vi "refreshElements.vi"(8 "error in (no error)":errorcluster, 9 "settingsFrontEndEvents":T1, 10 "Tab ref in":refnum<vi>) -> (0 "error out":errorcluster, 2 "Tab ref out":refnum<vi>)   [LabVIEW 2009, in "Views.lvlib" / "Camera.lvlib" / "andorSettingsViewer.lvclass"]
uses:
  andorSettingsViewer.lvclass
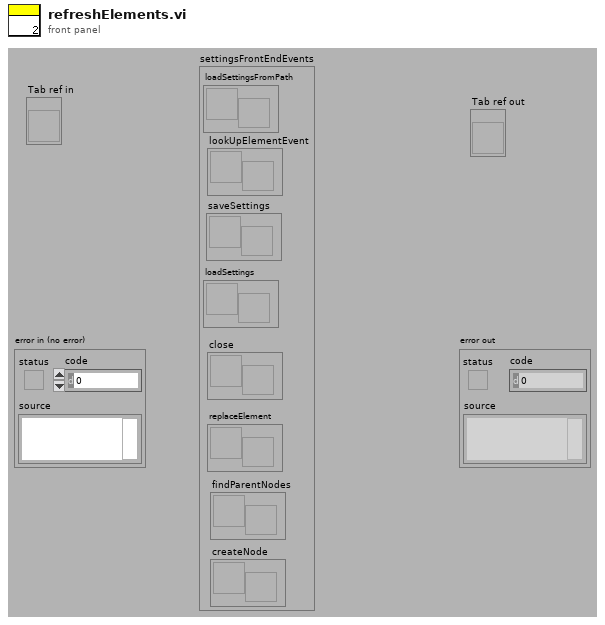
[diagram p1: front panel]
types:
  T1 = cluster{"loadSettingsFromPath":refnum<user-event>, "lookUpElementEvent":refnum<user-event>, "saveSettings":refnum<user-event>, "loadSettings":refnum<user-event>, "close":refnum<user-event>, "replaceElement":refnum<user-event>, "findParentNodes":refnum<user-event>, "createNode":refnum<user-event>}
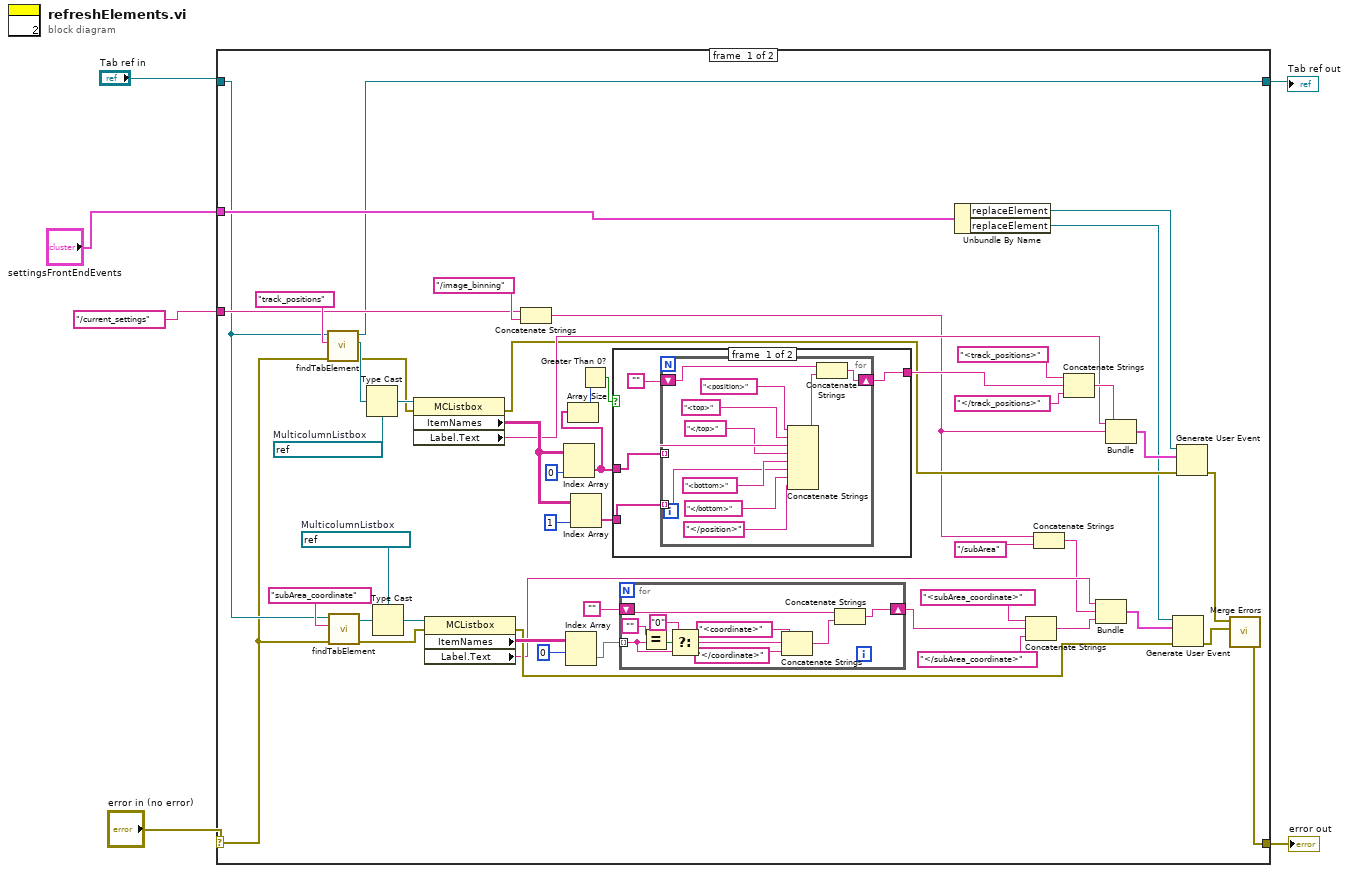
[diagram p0: block diagram]
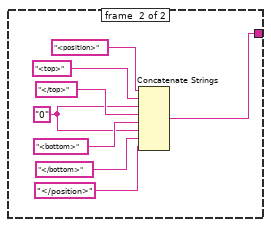
[diagram p2: hidden frame]
diagram:
  n1 = case shown="No Error" "error in (no error)" {
    selector: "error in (no error)" -> [w11 w90]
    tunnel: [w8 w90] -> w5
    tunnel: "Tab ref in" -> [w12 w89]
    tunnel: [w7 w89] -> w2
    tunnel: "settingsFrontEndEvents" -> [w16 _]
    tunnel: "/current_settings" -> [w13 _]
    frame #0 {
      w37 = refnum<vi> refnum  # MulticolumnListbox
      w42 = refnum<vi> refnum  # MulticolumnListbox
      n2 = call "findTabElement.vi"("error in (no error)"=w11, "replaceElementLabeled"="track_positions", "Tab ref in"=w12) -> ("error out"=w40:errorcluster, "Tab Control"=w44:refnum<vi>, "Tab ref out"=w7:refnum<vi>)  [unwired: 5 in, 1 out]
      n3 = call "findTabElement.vi"("error in (no error)"=w11, "replaceElementLabeled"="subArea_coordinate", "Tab ref in"=w12) -> ("error out"=w34:errorcluster, "Tab Control"=w36:refnum<vi>)  [unwired: 5 in, 2 out]
      n4 = Type Cast(type=w42, x=w44) -> (*(type *) &x=w43:refnum<vi>)
      n5 = Type Cast(type=w37, x=w36) -> (*(type *) &x=w35:refnum<vi>)
      n6 = property class="MCListbox"(reference=w43, error in=w40) -> (error out=w39:errorcluster, "ItemNames"=w54:string[][], "Label.Text"=w45:string)  [unwired: 1 out]
      n7 = property class="MCListbox"(reference=w35, error in=w34) -> (error out=w26:errorcluster, "ItemNames"=w33:string[][], "Label.Text"=w25:string)  [unwired: 1 out]
      n8 = Concatenate Strings(w13, "/image_binning") -> (w23:string)
      n9 = Index Array(array=w54, index (col)=0) -> (element=w17:string[])  [unwired: 1 in]
      n10 = Index Array(array=w33, index (row)=0) -> (element=w31:string[])  [unwired: 1 in]
      n11 = Array Size(array=w17) -> (size(s)=w18:i32)
      n12 = Index Array(array=w54, index (col)=1) -> (element=w52:string[])  [unwired: 1 in]
      n13 = Greater Than 0?(x=w18) -> (x > 0?=w19:bool)
      n14 = case shown="False" w19 {
        tunnel: w17 -> [w59 _]
        tunnel: w52 -> [w58 _]
        tunnel: [w56 w72] -> w50
        frame #0 {
          n15 = for {
            tunnel: w59 -> [w68] mode=indexing
            tunnel: w58 -> [w65] mode=indexing
            shift-right: [w60] -> w56
            shift-left: "" -> [w62]
            n16 = Concatenate Strings("<position>", "<top>", w68, "</top>", "<bottom>", w65, "</bottom>", "</position>") -> (w61:string)
            n17 = Concatenate Strings(w62, w61) -> (w60:string)
          }
        }
        frame #1 {
          w71 = "0"
          n18 = Concatenate Strings("<position>", "<top>", w71, "</top>", "<bottom>", w71, "</bottom>", "</position>") -> (w72:string)
        }
      }
      n19 = for {
        tunnel: w31 -> [w80] mode=indexing
        shift-right: [w86] -> w27
        shift-left: "" -> [w85]
        n20 = Equal?(x="", y=w80) -> (x = y?=w82:bool)
        n21 = Select(t="0", s=w82, f=w80) -> (s? t:f=w79:string)
        n22 = Concatenate Strings("<coordinate>", w79, "</coordinate>") -> (w84:string)
        n23 = Concatenate Strings(w85, w84) -> (w86:string)
      }
      n24 = Unbundle By Name(w16) -> ("replaceElement"=w15:refnum<user-event>, "replaceElement"=w14:refnum<user-event>)
      n25 = Concatenate Strings("<subArea_coordinate>", w27, "</subArea_coordinate>") -> (w24:string)
      n26 = Concatenate Strings(w23, "/subArea") -> (w21:string)
      n27 = Concatenate Strings("<track_positions>", w50, "</track_positions>") -> (w47:string)
      n28 = Bundle("Label.Text"=w25, w21, w24) -> (w20:cluster{"Label.Text":string, string, string})  [unwired: 1 in]
      n29 = Bundle("Label.Text"=w45, w23, w47) -> (w46:cluster{"Label.Text":string, string, string})  [unwired: 1 in]
      n30 = Generate User Event(user event=w14, event data cluster=w20, error in=w26) -> (error out=w9:errorcluster)  [unwired: 1 out]
      n31 = Generate User Event(user event=w15, event data cluster=w46, error in=w39) -> (error out=w10:errorcluster)  [unwired: 1 out]
      n32 = call <vilib>:"Merge Errors.vi"("error in 2 (no error)"=w9, "error in 1 (no error)"=w10) -> ("error out"=w8:errorcluster)  [unwired: 5 in]
    }
    frame #1 {
    }
  }
  "error out" <- w5
  "Tab ref out" <- w2
